vi "Destroy.vi"(8 "error in (no error)":errorcluster, 11 "Planet in":refnum<class "Planet.lvclass">) -> (0 "error out":errorcluster)   [LabVIEW 2015, in "Planet.lvclass"]
uses:
  Planet.lvclass
  Planet.lvclass/Planet.ctl
  Resource Manager/Resource Manager.lvclass
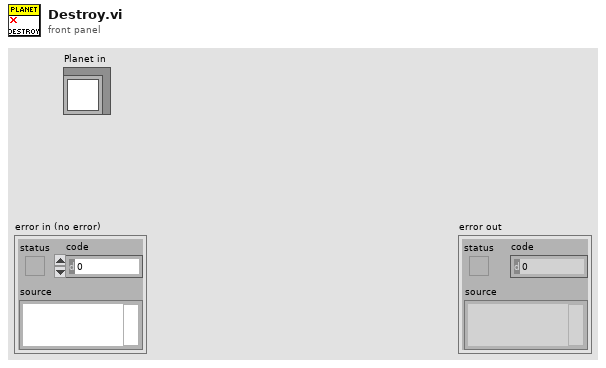
[diagram p1: front panel]
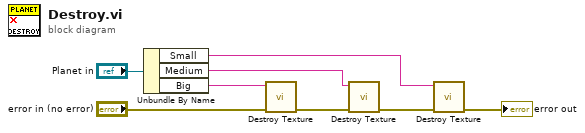
[diagram p0: block diagram]
diagram:
  n1 = Unbundle By Name("Planet in") -> ("Small"=w1:string, "Medium"=w2:string, "Big"=w6:string)
  n2 = call "Destroy Texture.vi"("error in (no error)"="error in (no error)", "Texture Name"=w6) -> ("error out"=w5:errorcluster)  [unwired: 9 in]
  n3 = call "Destroy Texture.vi"("error in (no error)"=w5, "Texture Name"=w2) -> ("error out"=w4:errorcluster)  [unwired: 9 in]
  n4 = call "Destroy Texture.vi"("error in (no error)"=w4, "Texture Name"=w1) -> ("error out"=→"error out":errorcluster)  [unwired: 9 in]
